vi "RampDown.vi"(2 "Current for Gravity compensation":dbl, 3 "Position [deg]":dbl, 4 "Target Position [deg]":dbl) -> (0 "CurrentOut [A]":dbl, 1 "Boolean":bool)   [LabVIEW 2019]
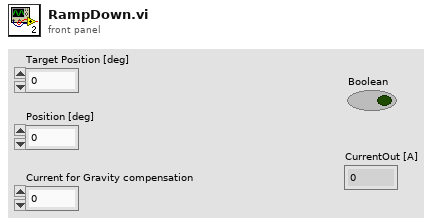
[diagram p1: front panel]
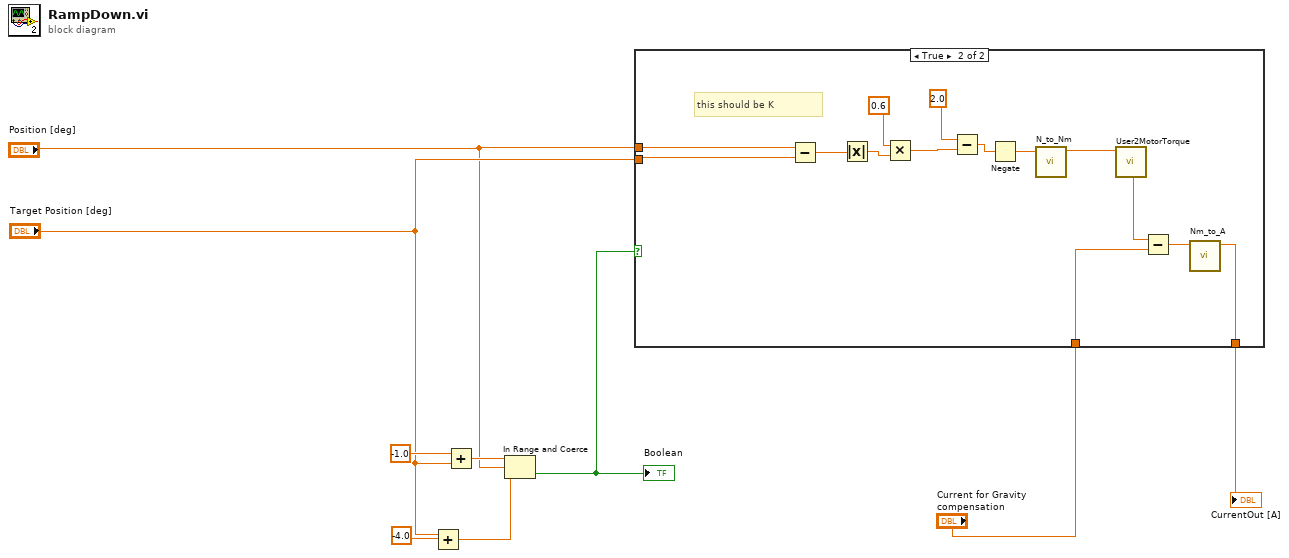
[diagram p0: block diagram]
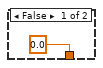
[diagram p2: hidden frame]
diagram:
  n1 = Add(x="Target Position [deg]", y=-4.0) -> (x+y=w5:dbl)
  n2 = Add(x=-1.0, y="Target Position [deg]") -> (x+y=w6:dbl)
  n3 = In Range and Coerce(upper limit=w6, x="Position [deg]", lower limit=w5) -> (In Range?=w9:bool)  [unwired: 1 out]
  "Boolean" <- w9
  n4 = case shown="True" w9 {
    tunnel: [0.0 ("u") w23] -> w3
    tunnel: "Current for Gravity compensation" -> [_ w22]
    tunnel: "Target Position [deg]" -> [_ w18]
    tunnel: "Position [deg]" -> [_ w19]
    frame False {
    }
    frame True {
      # "this should be K"
      n5 = Subtract(x=w19, y=w18) -> (x-y=w17:dbl)
      n6 = Absolute Value(x=w17) -> (abs(x)=w15:dbl)
      n7 = Multiply(x=0.6, y=w15) -> (x*y=w12:dbl)
      n8 = Subtract(x=2.0, y=w12) -> (x-y=w11:dbl)
      n9 = Negate(x=w11) -> (-x=w14:dbl)
      n10 = call "N_to_Nm.vi"("Force [N]"=w14) -> ("Torque [Nm]"=w24:dbl)  [unwired: 10 in]
      n11 = call "User2MotorTorque.vi"("User Torque [Nm]"=w24) -> ("Motor Torque [Nm]"=w20:dbl)  [unwired: 10 in]
      n12 = Subtract(x=w20, y=w22) -> (x-y=w21:dbl)
      n13 = call "Nm_to_A.vi"("Torque [Nm]"=w21) -> ("Current [A]"=w23:dbl)  [unwired: 10 in]
    }
  }
  "CurrentOut [A]" <- w3
